vi "Parse_response.vi"(8 "error in (no error)":errorcluster, 11 "Response in":refnum<class "Response.lvclass">) -> (0 "error out":errorcluster, 3 "Response out":refnum<class "Response.lvclass">)   [LabVIEW 2016, in "Response.lvclass"]
uses:
  Response.lvclass
  Response.lvclass/Response.ctl
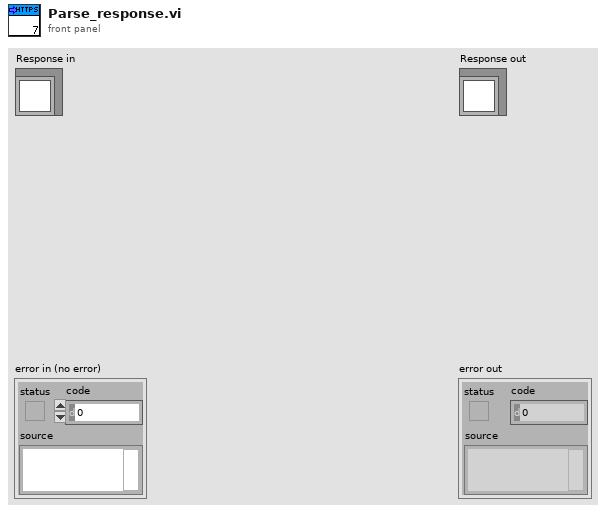
[diagram p1: front panel]
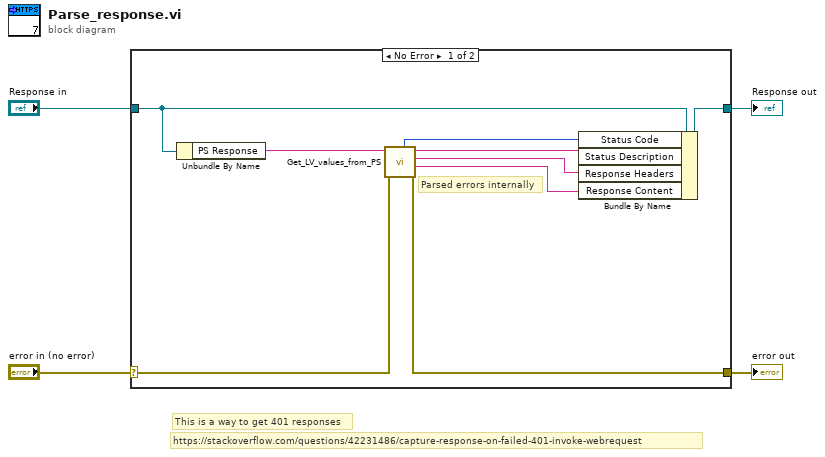
[diagram p0: block diagram]
diagram:
  # "This is a way to get 401 responses"
  # "https://stackoverflow.com/questions/42231486/capture-response-on-failed-401-invoke-webrequest"
  n1 = case shown="No Error" "error in (no error)" {
    selector: "error in (no error)" -> [w10 w15]
    tunnel: [w9 w15] -> w3
    tunnel: [w12 w14] -> w1
    tunnel: "Response in" -> [w13 w14]
    frame No Error {
      # "Parsed errors internally"
      n2 = Unbundle By Name(w13) -> ("PS Response"=w11:string)
      n3 = call "Get_LV_values_from_PS.vi"("error in (no error)"=w10, "Response"=w11) -> ("error out"=w9:errorcluster, "Content"=w6:string, "Headers"=w7:string, "Status Description"=w8:string, "Status Code"=w5:i32)  [unwired: 4 in, 1 out]
      n4 = Bundle By Name(cluster=w13, "Status Code"=w5, "Status Description"=w8, "Response Headers"=w7, "Response Content"=w6) -> (w12:refnum<class "Response.lvclass">)
    }
    frame Error {
    }
  }
  "error out" <- w3
  "Response out" <- w1
